vi "ma_Sort extacted tones by amplitude.vi"(4 "extracted tones in":T1(array[cluster]) {"phase [degree]" format="%.2f"; "amplitude" format="%.4f"; "frequency [Hz]" format="%.2f"}) -> (1 "extracted tones (sorted by amplitude)":T1(array[cluster]) {"phase [degree]" format="%.2f"; "amplitude" format="%.4f"; "frequency [Hz]" format="%.2f"})   [LabVIEW 2020, in "NI_MAPro.lvlib"]
uses:
  NI_MAPro.lvlib
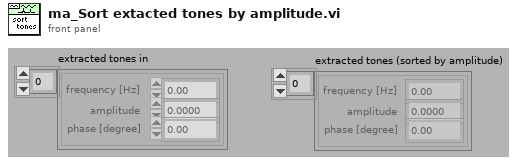
[diagram p1: front panel]
types:
  T1 = cluster{"frequency [Hz]":dbl, "amplitude":dbl, "phase [degree]":dbl}[]
  T2 = cluster{"frequency [Hz]":dbl, "amplitude":dbl, "phase [degree]":dbl}
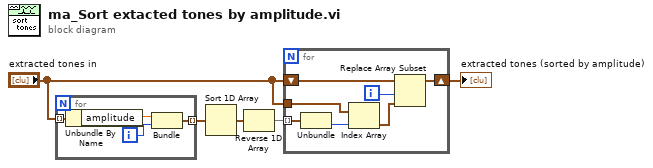
[diagram p0: block diagram]
diagram:
  n1 = for {
    tunnel: "extracted tones in" -> [w9] mode=indexing
    tunnel: [w6] -> w5 mode=indexing
    i -> [w7]
    n2 = Unbundle By Name(w9) -> ("amplitude"=w8:dbl)
    n3 = Bundle("amplitude"=w8, w7) -> (w6:cluster{"amplitude":dbl, i32})  [unwired: 1 out]
  }
  n4 = Sort 1D Array(array=w5) -> (sorted array=w4:cluster{"amplitude":dbl, i32}[])
  n5 = Reverse 1D Array(array=w4) -> (reversed array=w1:cluster{"amplitude":dbl, i32}[])
  n6 = for {
    shift-right: [w12] -> w2
    shift-left: "extracted tones in" -> [w13]
    tunnel: w1 -> [w16] mode=indexing
    tunnel: "extracted tones in" -> [w14]
    i -> [w11]
    n7 = Unbundle(w16) -> (w15:i32)  [unwired: 1 out]
    n8 = Index Array(array=w14, index=w15) -> (element=w10:T2)
    n9 = Replace Array Subset(array=w13, new element=w10, index=w11) -> (w12:T1)
  }
  "extracted tones (sorted by amplitude)" <- w2
